vi "Encrypt (Public Key Bytes).vi"(7 "Padding Mode":T1=enum."OaepSHA512", 8 "error in (no error)":errorcluster, 10 "Raw data in":u8[](array[numeric]), 11 "Public key in":u8[](array[numeric])) -> (0 "error out":errorcluster, 2 "Encrypted data out":u8[](array[numeric]))   [LabVIEW 2021, in "dotNET Crypto Asymmetric Encryption.lvlib"]
doc: "Encrypt data using the public key. This can only be decrypted using the corresponding private key."
uses:
  dotNET Crypto Asymmetric Encryption.lvlib
  RSAEncryptionPadding.ctl
  System.Core
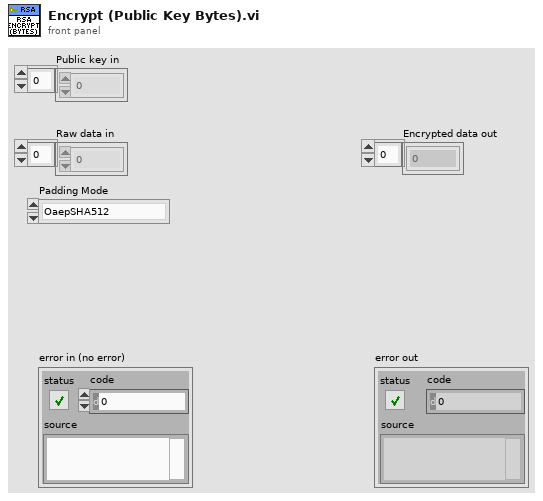
[diagram p1: front panel]
types:
  T1 = typedef "dotNET Crypto Asymmetric Encryption.lvlib/RSAEncryptionPadding.ctl" = enum16{"OaepSHA1", "OaepSHA256", "OaepSHA384", "OaepSHA512", "Pkcs1"}
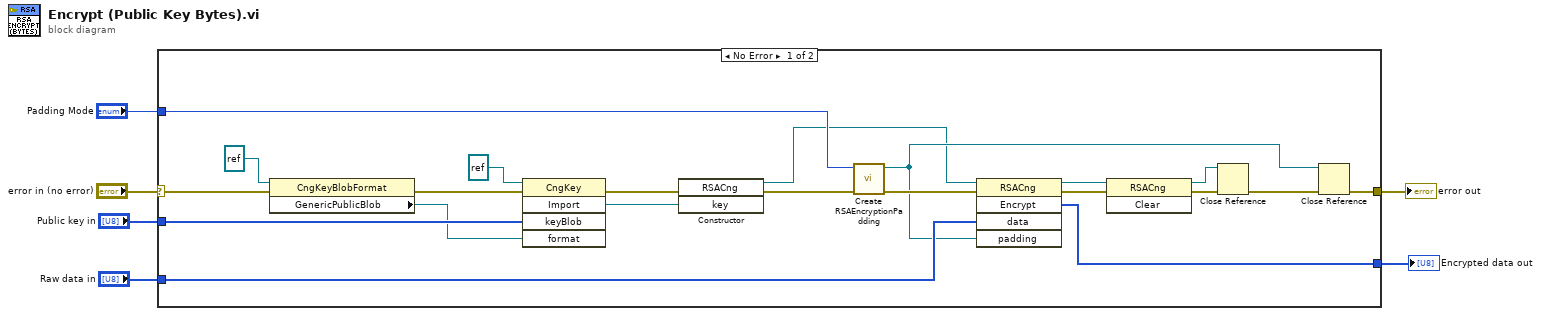
[diagram p0: block diagram]
diagram:
  n1 = case shown="No Error" "error in (no error)" {
    selector: "error in (no error)" -> [w9 w28]
    tunnel: "Raw data in" -> [w27 _]
    tunnel: [w26 _] -> w5
    tunnel: "Padding Mode" -> [w19 _]
    tunnel: [w16 w28] -> w3
    tunnel: "Public key in" -> [w12 _]
    frame No Error {
      n2 = property class="CngKeyBlobFormat"(reference=refnum<k24> refnum ("format"), error in=w9) -> (error out=w8:errorcluster, "GenericPublicBlob"=w7:refnum<k24>)  [unwired: 1 out]
      n3 = invoke class="CngKey" method="Import"(reference=refnum<k24> refnum, error in=w8, "keyBlob"=w12, "format"=w7) -> (error out=w13:errorcluster, "Import"=w11:refnum<k24>)  [unwired: 1 in, 3 out]
      n4 = constructor class="RSACng"(error in=w13, "key"=w11) -> (reference out=w15:refnum<k24>, error out=w20:errorcluster)  [unwired: 2 in, 2 out]
      n5 = call "Create RSAEncryptionPadding.vi"("error in (no error)"=w20, "Padding Mode"=w19) -> ("error out"=w18:errorcluster, "RSAEncryptionPadding"=w17:refnum<k24>)  [unwired: 8 in]
      n6 = invoke class="RSACng" method="Encrypt"(reference=w15, error in=w18, "data"=w27, "padding"=w17) -> (reference out=w24:refnum<k24>, error out=w25:errorcluster, "Encrypt"=w26:u8[])  [unwired: 1 in, 2 out]
      n7 = invoke class="RSACng" method="Clear"(reference=w24, error in=w25) -> (reference out=w22:refnum<k24>, error out=w21:errorcluster)  [unwired: 1 in, 1 out]
      n8 = Close Reference(reference=w22, error in (no error)=w21) -> (error out=w23:errorcluster)
      n9 = Close Reference(reference=w17, error in (no error)=w23) -> (error out=w16:errorcluster)
    }
    frame Error {
    }
  }
  "error out" <- w3
  "Encrypted data out" <- w5
